vi "TEC Server.vi"(11 "DVR In":refnum<data-value>) -> (3 "DVR Out":refnum<data-value>)   [LabVIEW 2015]
uses:
  Data/Nicholas Data.lvclass
  Session/Raw FPGA/FPGA Session.lvclass
  Reusable/Session Log/System Log.lvclass
  Reusable/Session APIs/File Access/Config Data/Config Data.lvclass
  Session/FPGA Serial Session.lvclass
  Reusable/Session Log/System Log.lvclass/System Log.ctl
  Reusable/Session APIs/File Access/Config Data/Config Data.lvclass/Config Data.ctl
  Devices/TE Cooler/TE Cooler.lvclass
  Session/FPGA Serial Session.lvclass/FPGA Serial Session.ctl
  Reusable/Session APIs/Text Communication/Text Device Session.lvclass/Text Device Session.ctl
  Devices/Configurable Device/Configurable Device.lvclass/Configurable Device.ctl
  Devices/TE Cooler/TE Cooler.lvclass/TE Cooler.ctl
  Devices/TE Cooler/Data/TECData.lvclass
  Data/Nicholas Data.lvclass/Nicholas Data.ctl
  Session/Write fpgaSession.vi
  Reusable/Session APIs/Text Communication/Write hSysLog.vi
  Session/Write Timeout (ms).vi
  Devices/Configurable Device/Write Handle.vi
  Devices/TE Cooler/Write hSession.vi
  Devices/TE Cooler/Write Pad Read.vi
  Devices/TE Cooler/Write ID.vi
  Data/Write TE Data.vi
  Reusable/Session Log/Accessors/Write Main Path.vi
  Reusable/Session APIs/File Access/Config Data/Accessors/Write Cfg Path.vi
  <userlib>/_Session Fwk/Session - Root.lvclass
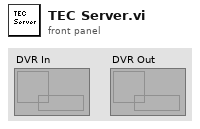
[diagram p1: front panel]
types:
  T1 = cluster{"Read Access":enum8{"Allowed", "Required", "None"}, "Write Access":enum8{"Allowed", "Required", "None"}}
  T2 = typedef "Session - Root.lvclass/Session Handle.ctl" = refnum<data-value>
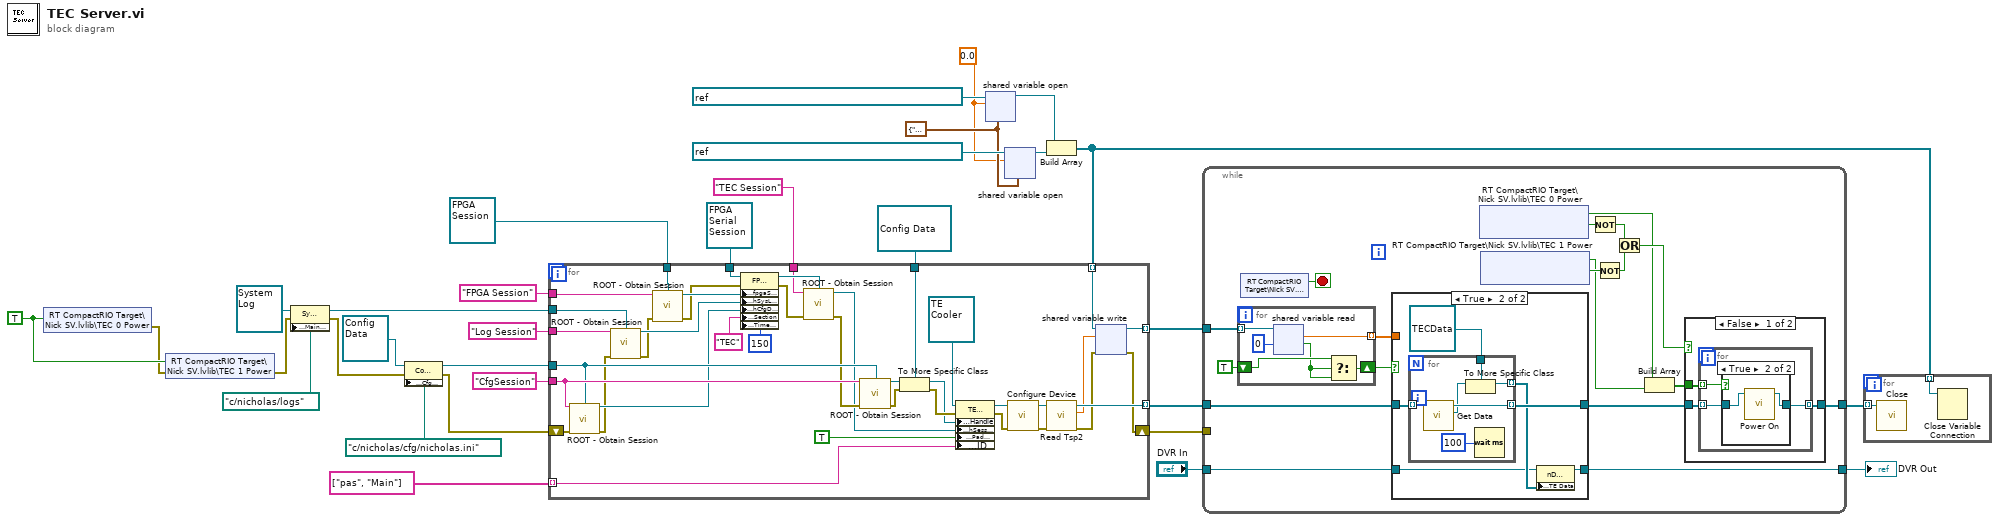
[diagram p0: block diagram]
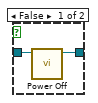
[diagram p2: hidden frame]
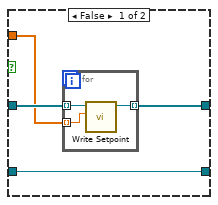
[diagram p4: hidden frame]
diagram:
  w6 = TRUE
  w11 = sgl 0.0 ("Tsp 0")
  w12 = T1 {"Read Access"=enum."Allowed", "Write Access"=enum."Allowed"} ("access")
  n1 = shared-variable "RT CompactRIO Target\\Nick SV.lvlib\\TEC 0 Power"(w6) -> (error out=w2:errorcluster)  [unwired: 1 in]
  n2 = shared-variable "RT CompactRIO Target\\Nick SV.lvlib\\TEC 1 Power"(w6, error in=w2) -> (error out=w1:errorcluster)
  n3 = property class="Sys Log"(reference=refnum<class "System Log.lvclass"> refnum ("Sys Log"), error in=w1, "Accessors:Main Path"=path "c:/nicholas/logs" ("Main Path")) -> (reference out=w20:refnum<class "System Log.lvclass">, error out=w4:errorcluster)
  n4 = property class="Config Data"(reference=refnum<class "Config Data.lvclass"> refnum ("Config Data"), error in=w4, "Accessors:Cfg Path"=path "c:/nicholas/cfg/nicholas.ini" ("Cfg Path")) -> (reference out=w21:refnum<class "Config Data.lvclass">, error out=w3:errorcluster)
  n5 = shared-variable-open(refnum<k21> "ni.var.psp://rt compactrio target/Nick SV/Tsp 0" ("shared variable refnum in"), w11, w12) -> (w10:refnum<k21>)  [unwired: 1 in, 1 out]
  n6 = shared-variable-open(refnum<k21> "ni.var.psp://rt compactrio target/Nick SV/Tsp 1" ("shared variable refnum in"), w11, w12) -> (w9:refnum<k21>)  [unwired: 1 in, 1 out]
  n7 = Build Array(w10, w9) -> (w7:refnum<k21>[])
  n8 = for {
    tunnel: w20 -> [w71]
    tunnel: "Log Session" ("Session Name ()") -> [w70]
    tunnel: refnum<class "FPGA Session.lvclass"> refnum ("FPGA Session") -> [w69]
    tunnel: "FPGA Session" ("Session Name ()") -> [w68]
    tunnel: w21 -> [w58]
    tunnel: "CfgSession" ("Session Name ()") -> [w59]
    tunnel: refnum<class "FPGA Serial Session.lvclass"> refnum ("FPGA Serial Session.lvclass") -> [w66]
    tunnel: [w54] -> w17 mode=indexing
    tunnel: refnum<data-value> refnum ("Session Handle") -> [w61]
    tunnel: "TEC Session" ("Session Name ()") -> [w60]
    tunnel: string[] ["pas", "Main"] -> [w37] mode=indexing
    tunnel: w7 -> [w53] mode=indexing
    tunnel: [w49] -> w8 mode=indexing
    shift-right: [w50] -> w5
    shift-left: w3 -> [w33]
    n9 = call <userlib>:"ROOT - Obtain Session.vi"("Session Name ()"=w59, "OBJ - Session"=w58, "error in (no error)"=w33) -> ("Session Handle"=w57:T2, "error out"=w34:errorcluster)  [unwired: 10 in, 1 out]
    n10 = call <userlib>:"ROOT - Obtain Session.vi"("Session Name ()"=w70, "OBJ - Session"=w71, "error in (no error)"=w34) -> ("Session Handle"=w64:T2, "error out"=w35:errorcluster)  [unwired: 10 in, 1 out]
    n11 = call <userlib>:"ROOT - Obtain Session.vi"("Session Name ()"=w68, "OBJ - Session"=w69, "error in (no error)"=w35) -> ("Session Handle"=w67:T2, "error out"=w36:errorcluster)  [unwired: 10 in, 1 out]
    n12 = property class="FPGA Serial Session"(reference=w66, error in=w36, "Accessors:fpgaSession"=w67, "Accessors:hSysLog"=w64, "Accessors:hCfgData"=w57, "Accessors:Section"="TEC" ("Section"), "Accessors:Timeout (ms)"=150 ("Timeout (ms)")) -> (reference out=w65:refnum<class "FPGA Serial Session.lvclass">, error out=w63:errorcluster)
    n13 = call <userlib>:"ROOT - Obtain Session.vi"("Session Name ()"=w60, "OBJ - Session"=w65, "error in (no error)"=w63) -> ("Session Handle"=w40:T2, "error out"=w48:errorcluster)  [unwired: 10 in, 1 out]
    n14 = call <userlib>:"ROOT - Obtain Session.vi"("Session Name ()"=w59, "OBJ - Session"=w58, "error in (no error)"=w48) -> ("Session Handle"=w62:T2, "error out"=w44:errorcluster)  [unwired: 10 in, 1 out]
    n15 = To More Specific Class(target class=w61, reference=w62, error in=w44) -> (specific class reference=w42:refnum<data-value>, error out=w43:errorcluster)
    n16 = property class="TE Cooler"(reference=refnum<class "TE Cooler.lvclass"> refnum ("TE Cooler.lvlib:TE Cooler"), error in=w43, "Accessors:Handle"=w42, "Accessors:hSession"=w40, "Accessors:Pad Read"=TRUE ("Pad Read"), "Accessors:ID"=w37) -> (reference out=w46:refnum<class "TE Cooler.lvclass">, error out=w45:errorcluster)
    n17 = call-dynamic "Configure Device.vi"("error in"=w45, "TE Cooler in"=w46) -> ("error out"=w55:errorcluster, "TE Cooler out"=w56:refnum<class "TE Cooler.lvclass">)  [unwired: 8 in]
    n18 = call "Read Tsp2.vi"("error in (no error)"=w55, "TE Cooler in"=w56) -> ("error out"=w51:errorcluster, "Tsp"=w52:sgl, "TE Cooler out"=w54:refnum<class "TE Cooler.lvclass">)  [unwired: 7 in]
    n19 = shared-variable-write(w53, w51, w52) -> (w49:refnum<k21>, w50:errorcluster)
  }
  n20 = while {
    tunnel: [w72] -> w25
    tunnel: w17 -> [w88]
    tunnel: "DVR In" -> [w87]
    tunnel: [w86] -> w15
    tunnel: w8 -> [w85]
    tunnel: w5 -> [_]
    stop <- w89 stop-if-true
    n21 = for {
      tunnel: w85 -> [w106] mode=indexing
      tunnel: [w104] -> w83 mode=indexing
      shift-right: [w101] -> w82
      shift-left: TRUE -> [w103]
      n22 = shared-variable-read(w106, 0 ("timeout ms")) -> (w102:bool, w104:sgl)  [unwired: 1 in, 3 out]
      n23 = Select(t=w103, s=w102, f=w102) -> (s? t:f=w101:bool)
    }
    n24 = shared-variable "RT CompactRIO Target\\Nick SV.lvlib\\Stop"() -> (w89:bool)  [unwired: 1 in, 1 out]
    n25 = case shown="True" w82 {
      tunnel: [w110 w119] -> w77
      tunnel: w88 -> [w108 w116]
      tunnel: w87 -> [w109 w115]
      tunnel: [w109 w114] -> w86
      tunnel: w83 -> [w107 _]
      frame False {
        n26 = for {
          tunnel: [w113] -> w110 mode=indexing
          tunnel: w107 -> [w112] mode=indexing
          tunnel: w108 -> [w111] mode=indexing
          n27 = call "Write Setpoint.vi"("SP"=w112, "TE Cooler in"=w111) -> ("TE Cooler out"=w113:refnum<class "TE Cooler.lvclass">)  [unwired: 8 in, 1 out]
        }
      }
      frame True {
        n28 = for {
          tunnel: [w125] -> w119 mode=indexing
          tunnel: refnum<class "TECData.lvclass"> refnum ("TE Cooler.lvlib:TEC Data") -> [w123]
          tunnel: [w122] -> w117 mode=indexing
          tunnel: w116 -> [w121] mode=indexing
          n29 = call-dynamic "Get Data.vi"("Cfg Dev in"=w121) -> ("Data"=w124:refnum<class "Data.lvclass">, "Cfg Dev out"=w125:refnum<class "TE Cooler.lvclass">)  [unwired: 8 in, 1 out]
          n30 = To More Specific Class(target class=w123, reference=w124) -> (specific class reference=w122:refnum<class "TECData.lvclass">)  [unwired: 1 in, 1 out]
          n31 = Wait (ms)(milliseconds to wait=u32 100) -> ()  [unwired: 1 out]
        }
        n32 = property class="nData"(reference=w115, "Accessors:TE Data"=w117) -> (reference out=w114:refnum<data-value>)  [unwired: 1 in, 1 out]
      }
    }
    n33 = shared-variable "RT CompactRIO Target\\Nick SV.lvlib\\TEC 0 Power"() -> (w75:bool, w81:bool)  [unwired: 2 in, 1 out]
    n34 = shared-variable "RT CompactRIO Target\\Nick SV.lvlib\\TEC 1 Power"() -> (w74:bool, w80:bool)  [unwired: 2 in, 1 out]
    n35 = Not(x=w81) -> (.not. x?=w78:bool)
    n36 = Not(x=w80) -> (.not. x?=w79:bool)
    n37 = Or(x=w78, y=w79) -> (x .or. y?=w76:bool)
    n38 = Build Array(w75, w74) -> (w73:bool[])
    n39 = case shown="False" w76 {
      tunnel: w77 -> [w92 w100]
      tunnel: w73 -> [w91 _]
      tunnel: [w90 w100] -> w72
      frame False {
        n40 = for {
          tunnel: w92 -> [w94] mode=indexing
          tunnel: w91 -> [w95] mode=indexing
          tunnel: [w93] -> w90 mode=indexing
          n41 = case shown="True" w95 {
            tunnel: w94 -> [w97 w99]
            tunnel: [w96 w98] -> w93
            frame False {
              n42 = call "Power Off.vi"("TE Cooler in"=w97) -> ("TE Cooler out"=w96:refnum<class "TE Cooler.lvclass">)  [unwired: 9 in, 1 out]
            }
            frame True {
              n43 = call "Power On.vi"("TE Cooler in"=w99) -> ("TE Cooler out"=w98:refnum<class "TE Cooler.lvclass">)  [unwired: 9 in, 1 out]
            }
          }
        }
      }
      frame True {
      }
    }
  }
  "DVR Out" <- w15
  n44 = for {
    tunnel: w25 -> [w127] mode=indexing
    tunnel: w7 -> [w126] mode=indexing
    n45 = call-dynamic "Close.vi"("Cfg Dev in"=w127) -> ()  [unwired: 9 in, 2 out]
    n46 = Close Variable Connection(11:w126) -> ()  [unwired: 1 in, 1 out]
  }
